vi "In Range Inclusive and Coerce Float.vi"(2 "Lower limit (-1)":dbl=-1.0 format="%.2f", 3 "X (0)":dbl format="%.2f", 4 "Upper limit (1)":dbl=1.0 format="%.2f") -> (0 "In range?":bool, 1 "Coerced X":dbl format="%.2f")   [LabVIEW 2017]
doc: "Anritsu LabVIEW Toolkit\n\nDetermines whether a value entered in X falls within a range specified by the upper limit and lower limit inputs and coerces the value to fall within the range. If a value entered in X is above the value entered in upper limit, In Range Inclusive and Coerce coerces X to the upper limit value. If a value entered in X is below the value entered in lower limit, In Range Inclusive and Coerce coerces x to the lower limit value.\n\nINPUTS\n X - value to compare and coerce.\n Upper limit, Lower limit - X must be between these limits or equal to one of them.\n\nOUTPUTS\n Coerced X - the nearest legal value to X (will equal X if X is in range).\n In range? - True if X is between or equal to the limits.\n\nThis VI is essentially the same as the LabVIEW 6i built-in function In Range & Coerce.vi, with the exception that this VI always includes the upper and lower limits and this VI can be correctly saved off in LabVIEW 5.0 format. If an application will be written in LabVIEW 6i and never stored in 5.0 format, it would be wiser to use the built-in functions."
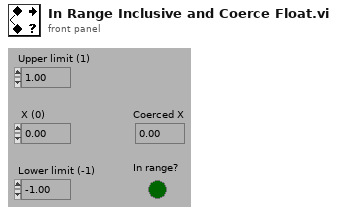
[diagram p1: front panel]
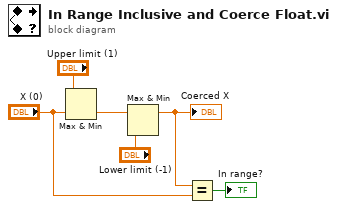
[diagram p0: block diagram]
diagram:
  n1 = Max & Min(x="Upper limit (1)", y="X (0)") -> (min(x,y)=w5:dbl)  [unwired: 1 out]
  n2 = Max & Min(x=w5, y="Lower limit (-1)") -> (max(x,y)=w2:dbl)  [unwired: 1 out]
  "Coerced X" <- w2
  n3 = Equal?(x=w2, y="X (0)") -> (x = y?=→"In range?":bool)
